vi "System check.vi"() -> (3 "Abort":bool)   [LabVIEW 2021]
doc: "Finds the NBMIO-16X board and the volume name.\nScott Hannahs, FBNML, Jan 1992"
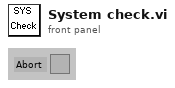
[diagram p1: front panel]
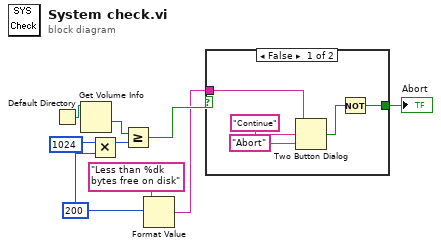
[diagram p0: block diagram]
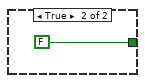
[diagram p2: hidden frame]
diagram:
  w4 = 200
  n1 = Default Directory() -> (w7:path)
  n2 = Get Volume Info(11:w7) -> (1:w8:i64)  [unwired: 1 in, 5 out]
  n3 = Multiply(x=1024, y=w4) -> (x*y=w3:i32)
  n4 = Greater Or Equal?(x=w8, y=w3) -> (x >= y?=w9:bool)
  n5 = Format Value(format string="Less than %dk bytes free on disk", value (0)=w4) -> (output string=w2:string)  [unwired: 1 in]
  n6 = case shown="False" w9 {
    tunnel: w2 -> [w12 _]
    tunnel: [w10 FALSE] -> w1
    frame False {
      n7 = Two Button Dialog(message=w12, 1:"Abort", 2:"Continue") -> (T button?=w11:bool)
      n8 = Not(x=w11) -> (.not. x?=w10:bool)
    }
    frame True {
    }
  }
  "Abort" <- w1
